vi "Export.vi"(8 "error in (no error)":errorcluster, 11 "strict-JUnit in":refnum<class "strict-JUnit.lvclass">) -> (0 "error out":errorcluster, 3 "strict-JUnit out":refnum<class "strict-JUnit.lvclass">)   [LabVIEW 2013, in "strict-JUnit.lvclass"]
uses:
  strict-JUnit.lvclass
  <vilib>/addons/_JKI Toolkits/Caraya/classes/Test Report/Test Report.lvclass
  <vilib>/addons/_JKI Toolkits/Caraya/classes/Test Result/Test Result.lvclass
  <vilib>/addons/_JKI Toolkits/Caraya/classes/Test Report.JUnit/Test Report.JUnit.lvclass
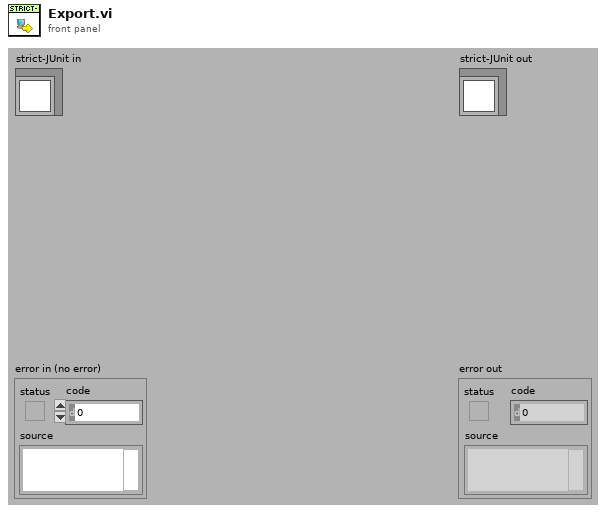
[diagram p1: front panel]
types:
  T1 = enum16{"open", "replace", "create", "open or create", "replace or create", "replace or create with confirmation"}
  T2 = typedef "Caraya.lvlib/Test Result.lvclass/Node Results.ctl" = cluster{"Node":T3, "Assertions":T5[]}
  T3 = typedef "Caraya.lvlib/Test Result.lvclass/Test Node.ctl" = cluster{"Test Registration":T4, "Defined":bool, "Passed":bool}
  T4 = typedef "Caraya.lvlib/Test Result.lvclass/Test Registration Data.ctl" = cluster{"Name":string, "Call Chain":string[], "Time Stamp":timestamp, "Test ID":string, "Caller ID":string}
  T5 = typedef "Caraya.lvlib/Test Result.lvclass/Assert Event Data.ctl" = cluster{"Name":string, "Passed":bool, "Call Chain":string[], "Test Error":errorcluster, "Time Stamp":timestamp, "Unique Assert ID":string, "Test ID":string, "Execution time (s)":dbl, "Verbose Explanation":string}
  T6 = typedef "Caraya.lvlib/Test Report.JUnit.lvclass/testcase -- cluster.ctl" = cluster{"classname":string, "name":string, "time":dbl, "skipped":bool, "failure":bool, "failure message":string, "failure description":string}
  T7 = typedef "Caraya.lvlib/Test Report.JUnit.lvclass/testsuite -- cluster.ctl" = cluster{"name":string, "errors":u32, "skipped":u32, "tests":u32, "failures":u32, "time":dbl, "timestamp":timestamp, "properties":T8[], "Call Chain":string[]}
  T8 = typedef "Caraya.lvlib/Test Report.JUnit.lvclass/property -- cluster.ctl" = cluster{"name":string, "value":string}
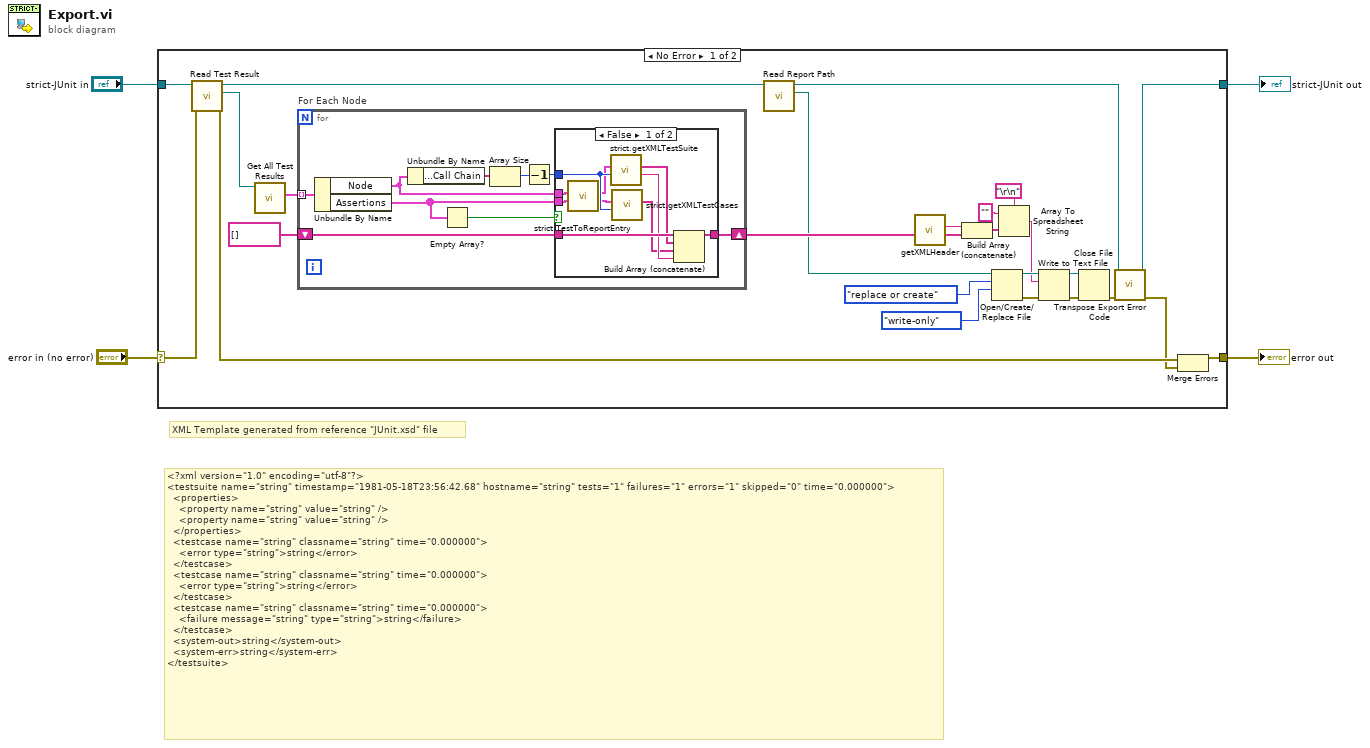
[diagram p0: block diagram]
diagram:
  # "XML Template generated from reference \"JUnit.xsd\" file"
  # "<?xml version=\"1.0\" encoding=\"utf-8\"?>\n<testsuite name=\"string\" timestamp=\"1981-05-18T23:56:42.68\" hostname=\"string\" tests=\"1\" failures=\"1\" errors=\"1\" skipped=\"0\" time=\"0.000000\">\n  <properties>\n    <property name=\"string\" value=\"string\" />\n    <property name=\"string\" value=\"string\" />\n  </properties>\n  <testcase name=\"string\" classname=\"string\" time=\"0.000000\">\n    <error type=\"string\">string</error>\n  </testcase>\n  <testcase name=\"string\" classname=\"string\" time=\"0.000000\">\n    <error type=\"string\">string</error>\n  </testcase>\n  <testcase name=\"string\" classname=\"string\" time=\"0.000000\">\n    <failure message=\"string\" type=\"string\">string</failure>\n  </testcase>\n  <system-out>string</system-out>\n  <system-err>string</system-err>\n</testsuite>"
  n1 = case shown="No Error" "error in (no error)" {
    selector: "error in (no error)" -> [w22 w51]
    tunnel: [w12 w51] -> w2
    tunnel: [w9 w50] -> w1
    tunnel: "strict-JUnit in" -> [w23 w50]
    frame No Error {
      n2 = call <vilib>:"Read Test Result.vi"("error in (no error)"=w22, "Test Report in"=w23) -> ("error out"=w13:errorcluster, "Caraya.lvlib:Test Result.lvclass"=w16:refnum<class "Test Result.lvclass">, "Test Report out"=w7:refnum<class "strict-JUnit.lvclass">)  [unwired: 7 in]
      n3 = call <vilib>:"Get All Test Results.vi"("Test Result in"=w16) -> ("Test Results"=w15:T2[])  [unwired: 8 in, 2 out]
      n4 = for "For Each Node" {
        shift-right: [w32] -> w14
        shift-left: string[] [] ("appended array") -> [w38]
        tunnel: w15 -> [w37] mode=indexing
        n5 = Unbundle By Name(w37) -> ("Node"=w35:T3, "Assertions"=w31:T5[])
        n6 = Unbundle By Name(w35) -> ("Test Registration.Call Chain"=w33:string[])
        n7 = Empty Array?(array=w31) -> (empty?=w34:bool)
        n8 = Array Size(array=w33) -> (size(s)=w36:i32)
        n9 = Decrement(x=w36) -> (x-1=w30:i32)
        n10 = case shown="False" w34 {
          tunnel: w35 -> [w42 _]
          tunnel: w31 -> [w41 _]
          tunnel: w38 -> [w48 w49]
          tunnel: [w47 w49] -> w32
          tunnel: w30 -> [w44 _]
          frame False {
            n11 = call "strict.TestToReportEntry.vi"("Asserts (aka. Test Cases)"=w41, "Node (aka. Test Suite)"=w42) -> ("testcases"=w39:T6[], "testsuite"=w40:T7)  [unwired: 7 in, 1 out]
            n12 = call "strict.getXMLTestSuite.vi"("indent level"=w44, "testsuite"=w40) -> ("testsuite (end)"=w45:string, "testsuite (start)"=w46:string[])  [unwired: 8 in]
            n13 = call "strict.getXMLTestCases.vi"("indent level"=w44, "testcases"=w39) -> ("XML testcases"=w43:string[])  [unwired: 9 in]
            n14 = Build Array (concatenate)(w48, w46, w43, w45) -> (w47:string[])
          }
          frame True {
          }
        }
      }
      n15 = call <vilib>:"Read Report Path.vi"("Test Report.JUnit in"=w7) -> ("Report Path"=w8:path, "Test Report.JUnit out"=w6:refnum<class "strict-JUnit.lvclass">)  [unwired: 9 in]
      n16 = call <vilib>:"getXMLHeader.vi"() -> ("xml header"=w5:string)  [unwired: 11 in]
      n17 = Build Array (concatenate)(w5, w14) -> (w20:string[])
      n18 = Open/Create/Replace File(file path (use dialog)=w8, operation (0:open)=T1."replace or create", access (0:read/write)=enum16{"read/write", "read-only", "write-only"}."write-only") -> (refnum out=w27:refnum<file>, error out=w26:errorcluster)  [unwired: 3 in, 1 out]
      n19 = Array To Spreadsheet String(delimiter (Tab)="\r\n", array=w20, 3:"" ("format string")) -> (spreadsheet string=w21:string)
      n20 = Write to Text File(file (use dialog)=w27, text=w21, error in=w26) -> (refnum out=w25:refnum<file>, error out=w24:errorcluster)  [unwired: 1 in, 1 out]
      n21 = Close File(refnum=w25, error in=w24) -> (error out=w11:errorcluster)  [unwired: 1 out]
      n22 = call-dynamic "Transpose Export Error Code.vi"("error in (no error)"=w11, "Test Report"=w6) -> ("error out"=w10:errorcluster, "Test Report out"=w9:refnum<class "strict-JUnit.lvclass">)  [unwired: 8 in]
      n23 = Merge Errors(w13, w10) -> (w12:errorcluster)
    }
    frame Error {
    }
  }
  "error out" <- w2
  "strict-JUnit out" <- w1
